vi "Center VI.vi"(8 "error in (no error)":errorcluster, 11 "VI Refnum":refnum<vi>) -> (0 "error out":errorcluster, 3 "VI Refnum Out":refnum<vi>)   [LabVIEW 2014]
doc: "<b>VI Type:</b> Standard VI \n<b>VI Description:</b> This VI will center the front panel and, if it's open, block diagram of the referenced VI on the primary monitor. \n<b>VI Version:</b> 1.0.Reviewed \n<b>Review Date:</b> 03/09/2012 \n<b>Author:</b> Jason Willis \n<b>Company:</b> BEI Precision System & Space Co. \n<b>Copyright:</b> Copyright © 2012 BEI Precision System & Space Co. \n<b>Dependencies:</b> None \n<b>Controls:</b> \n<b>Inputs:</b>\n<b>VI Refnum:</b>\nA refnum of the VI to be operated on\n\n<b>error in (no error):</b>\n<B>error in</B> can accept error information wired from VIs previously called. Use this information to decide if any functionality should be bypassed in the event of errors from other VIs.\n\nRight-click the <B>error in</B> control on the front panel and select <B>Explain Error</B> or <B>Explain Warning</B> from the shortcut menu for more information about the error. \n\n<b>Outputs:</b>\n<b>VI Refnum Out:</b>\nA refnum of the VI to be operated on\n\n<b>error out:</b>\n<B>error out</B> passes error or warning information out of a VI to be used by other VIs.\n\nRight-click the <B>error out</B> indicator on the front panel and select <B>Explain Error</B> or <B>Explain Warning</B> from the shortcut menu for more information about the error."
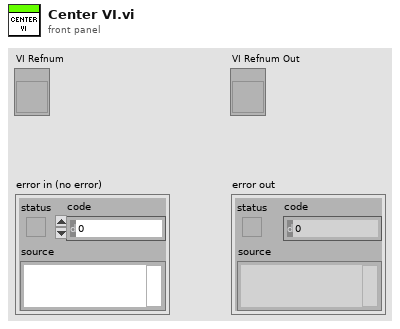
[diagram p1: front panel]
types:
  T1 = typedef "LVRectTypeDef.ctl" = cluster{"Left":i16, "Top":i16, "Right":i16, "Bottom":i16}
  T2 = enum32{"invalid VI type", "Standard VI", "Control VI", "Global VI", "Polymorphic VI", "Configuration VI", "SubSystem", "Facade VI", "Method VI", "Statechart Diagram VI"}
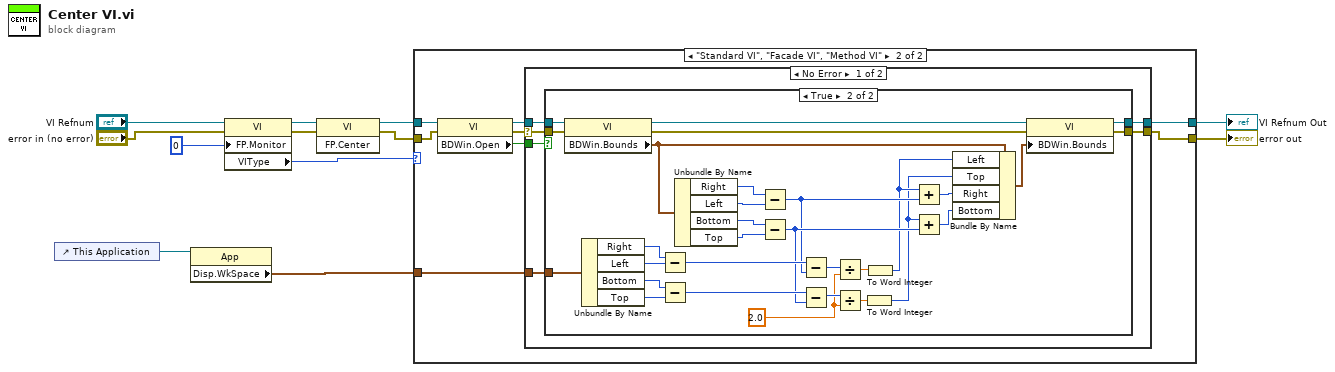
[diagram p0: block diagram]
diagram:
  n1 = control-ref of="This Application"() -> (w2:refnum<vi>)
  n2 = property class="App"(reference=w2) -> ("Disp.WkSpace"=w1:T1)  [unwired: 1 in, 2 out]
  n3 = property class="VI"(reference="VI Refnum", error in="error in (no error)", "FP.Monitor"=u16 0 ("Front Panel Window:Monitor")) -> (reference out=w5:refnum<vi>, error out=w6:errorcluster, "VIType"=w3:T2)
  n4 = invoke class="VI" method="FP.Center"(reference=w5, error in=w6) -> (reference out=w4:refnum<vi>, error out=w12:errorcluster)  [unwired: 1 in, 1 out]
  n5 = case shown="\"Standard VI\", \"Facade VI\", \"Method VI\"" w3 {
    tunnel: w12 -> [w14 w20]
    tunnel: [w13 w18] -> w10
    tunnel: [w14 w17] -> w7
    tunnel: w4 -> [w13 w16]
    tunnel: w1 -> [_ w15]
    frame "invalid VI type", Default {
    }
    frame "Standard VI", "Facade VI", "Method VI" {
      n6 = property class="VI"(reference=w16, error in=w20) -> (reference out=w19:refnum<vi>, error out=w22:errorcluster, "BDWin.Open"=w21:bool)
      n7 = case shown="No Error" w22 {
        selector: w22 -> [w26 w61]
        tunnel: w19 -> [w28 w62]
        tunnel: w21 -> [w27 _]
        tunnel: [w25 w62] -> w18
        tunnel: [w24 w61] -> w17
        tunnel: w15 -> [w23 _]
        frame No Error {
          n8 = case shown="True" w27 {
            tunnel: w26 -> [w29 w56]
            tunnel: w28 -> [w30 w57]
            tunnel: [w30 w50] -> w25
            tunnel: [w29 w49] -> w24
            tunnel: w23 -> [_ w48]
            frame False {
            }
            frame True {
              w36 = 2.0
              n9 = property class="VI"(reference=w57, error in=w56) -> (reference out=w54:refnum<vi>, error out=w55:errorcluster, "BDWin.Bounds"=w31:T1)
              n10 = Unbundle By Name(w48) -> ("Right"=w44:i16, "Left"=w47:i16, "Bottom"=w46:i16, "Top"=w45:i16)
              n11 = Subtract(x=w44, y=w47) -> (x-y=w42:i16)
              n12 = Subtract(x=w46, y=w45) -> (x-y=w41:i16)
              n13 = Unbundle By Name(w31) -> ("Right"=w58:i16, "Left"=w59:i16, "Bottom"=w60:i16, "Top"=w43:i16)
              n14 = Subtract(x=w58, y=w59) -> (x-y=w39:i16)
              n15 = Subtract(x=w60, y=w43) -> (x-y=w40:i16)
              n16 = Subtract(x=w42, y=w39) -> (x-y=w38:i16)
              n17 = Subtract(x=w41, y=w40) -> (x-y=w37:i16)
              n18 = Divide(x=w38, y=w36) -> (x/y=w35:dbl)
              n19 = Divide(x=w37, y=w36) -> (x/y=w34:dbl)
              n20 = To Word Integer(number=w34) -> (16bit integer=w32:i16)
              n21 = To Word Integer(number=w35) -> (16bit integer=w33:i16)
              n22 = Add(x=w33, y=w39) -> (x+y=w52:i16)
              n23 = Add(x=w32, y=w40) -> (x+y=w51:i16)
              n24 = Bundle By Name(cluster=w31, "Left"=w33, "Top"=w32, "Right"=w52, "Bottom"=w51) -> (w53:T1)
              n25 = property class="VI"(reference=w54, error in=w55, "BDWin.Bounds"=w53) -> (reference out=w50:refnum<vi>, error out=w49:errorcluster)
            }
          }
        }
        frame Error {
        }
      }
    }
  }
  "VI Refnum Out" <- w10
  "error out" <- w7
